vi "lsl create streaminfo.vi"(5 "source_id":string, 6 "channel_format":T1=2 items=["cft_float32"=1, "cft_double64"=2, "cft_string"=3, "cft_int32"=4, "cft_int16"=5, "cft_int8"=6, "cft_int64"=7, "cft_undefined"=0], 7 "samplingrate":dbl, 8 "error in (no error)":errorcluster, 9 "channel_count":i32=1, 10 "type":string="EEG", 11 "name":string="My EEG Device") -> (0 "error out":errorcluster, 3 "streaminfo":T2)   [LabVIEW 2016, in "Lab Streaming Layer.lvlib"]
doc: "extern LIBLSL_C_API lsl_streaminfo lsl_create_streaminfo(const char *name, const char *type, int32_t channel_count, double nominal_srate, lsl_channel_format_t channel_format, const char *source_id);"
uses:
  Lab Streaming Layer.lvlib
  Custom Controls/lsl_streaminfo.ctl
  Custom Controls/lsl_channel_format.ctl
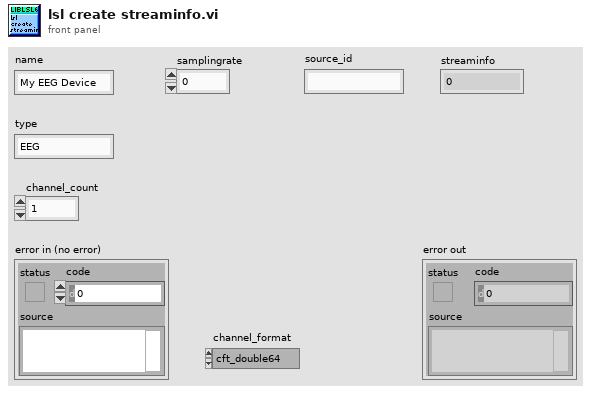
[diagram p1: front panel]
types:
  T1 = typedef "Lab Streaming Layer.lvlib/lsl_channel_format.ctl" = u32
  T2 = typedef "Lab Streaming Layer.lvlib/lsl_streaminfo.ctl" = u64
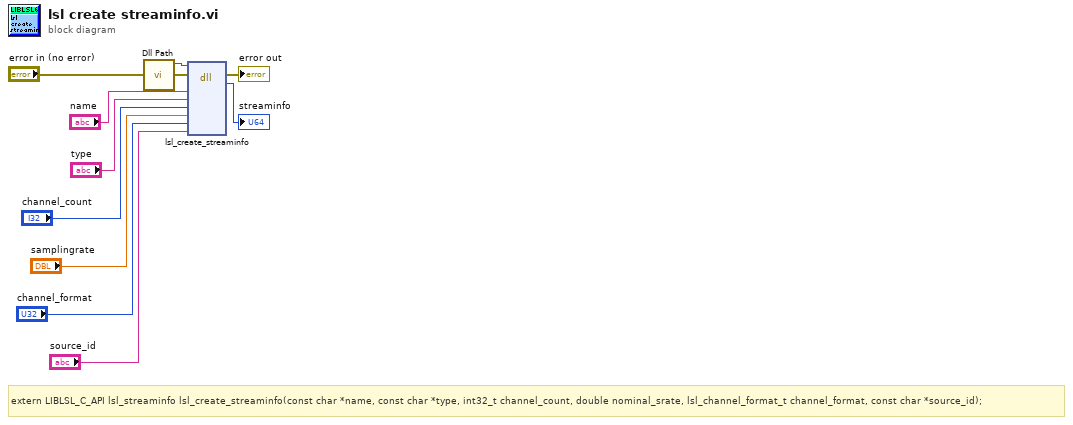
[diagram p0: block diagram]
diagram:
  # "extern LIBLSL_C_API lsl_streaminfo lsl_create_streaminfo(const char *name, const char *type, int32_t channel_count, double nominal_srate, lsl_channel_format_t channel_format, const char *source_id);"
  n1 = call "Dll Path.vi"() -> ("Dll path"=w1:path)  [unwired: 11 in]
  n2 = dll-call lib="E:/LabStreamingLayer/liblsl-LabVIEW-master/liblsl-LabVIEW-master/lsl.dll" fn="lsl_create_streaminfo"(path in=w1, error in="error in (no error)", "name"="name", "type"="type", "channel_count"="channel_count", "nominal_srate"="samplingrate", "channel_format"="channel_format", "source_id"="source_id") -> (error out=→"error out":errorcluster, "return type"=→"streaminfo":u64)  [unwired: 7 in, 1 out]
